vi "Close Window or Stop Actor Dialog.vi"(2 "Error In":errorcluster, 3 "Self Enqueuer":refnum<class "Message Enqueuer.lvclass">) -> (0 "Error Out":errorcluster)   [LabVIEW 2015, in "CS++Utilities.lvlib"]
doc: "Display a three button diolog to ask user whether to close window of stop actor."
uses:
  CS++Utilities.lvlib
  <vilib>/ActorFramework/Message Enqueuer/Message Enqueuer.lvclass
  Actors/CS++BaseActor Messages/Open Actor Core FP Msg/Open Actor Core FP Msg.lvclass/Open Actor Core FP Msg.ctl
  <vilib>/ActorFramework/Message Enqueuer/Message Enqueuer.lvclass/Message Enqueuer.ctl
  <vilib>/ActorFramework/Message Enqueuer/Enqueue.vi
  <vilib>/ActorFramework/Message Priority Queue/Priority Enqueue.vi
  Actors/CS++BaseActor Messages/Open Actor Core FP Msg/Open Actor Core FP Msg.lvclass
  <vilib>/ActorFramework/Stop Msg/Stop Msg.lvclass
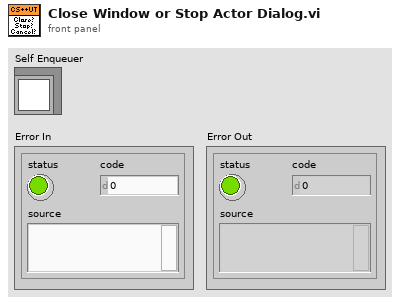
[diagram p1: front panel]
types:
  T1 = enum16{"Left Button", "Center Button", "Right Button", "Window Close"}
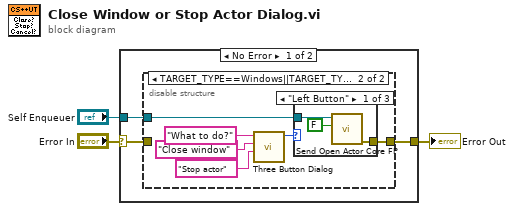
[diagram p0: block diagram]
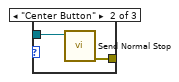
[diagram p3: hidden frame]
diagram:
  n1 = case shown="No Error" "Error In" {
    selector: "Error In" -> [w4 w19]
    tunnel: "Self Enqueuer" -> [w6 _]
    tunnel: [w5 w19] -> w2
    frame No Error {
      n2 = disable-structure shown="TARGET_TYPE==Windows||TARGET_TYPE==Unix||TARGET_TYPE==Mac" {
        disable-tunnel: w6 -> [_ w9]
        disable-tunnel: [w7 w8] -> w5
        disable-tunnel: w4 -> [w7 _]
        frame condition #0 {
        }
        frame condition #1 (active) {
          n3 = call <vilib>:"Three Button Dialog.vi"("Center Button Text (\"No\")"="Stop actor" ("Center Button Text (\"No\")"), "Left Button Text (\"Yes\")"="Close window" ("Left Button Text (\"Yes\")"), "message"="What to do?") -> ("Which Button?"=w13:T1)  [unwired: 8 in]
          n4 = case shown="\"Left Button\"" w13 {
            tunnel: [w15 w18 _] -> w8
            tunnel: w9 -> [w16 w17 _]
            frame "Left Button" {
              n5 = call "Send Open Actor Core FP.vi"("Open FP (F)"=FALSE, "Message Enqueuer"=w16) -> ("error out"=w15:errorcluster)  [unwired: 8 in, 1 out]
            }
            frame "Center Button" {
              n6 = call <vilib>:"Send Normal Stop.vi"("Message Enqueuer"=w17) -> ("error out"=w18:errorcluster)  [unwired: 10 in]
            }
            frame Default {
            }
          }
        }
      }
    }
    frame Error {
    }
  }
  "Error Out" <- w2
